vi "Display_ShowGameScreen.vi"(2 "Player":T1) -> ()   [LabVIEW 2018]
uses:
  TypDefs/Player_Enum.ctl
  <vilib>/Platform/TimedLoop/XDataNode/timing_clust.ctl
  <vilib>/Platform/TimedLoop/XDataNode/nitl_modes.ctl
  <vilib>/Platform/TimedLoop/XDataNode/wakeup.ctl
  <vilib>/rvi/Emulation/niFpgaSctlEmulationGetInTimedLoop.vi
  <vilib>/rvi/Emulation/niFpgaEmulationReportErrorSimple.vi
  <vilib>/rvi/Emulation/niFpgaGetClockAttributes.vi
  <vilib>/rvi/Emulation/niFpgaCriticalErrorInLSC.vi
  Control/Global_GameOver.vi
  <vilib>/Platform/TimedLoop/XDataNode/XDataNode.xnode
  <vilib>/Platform/TimedLoop/XDataNode/XDNodeRunTimeDep.lvlib
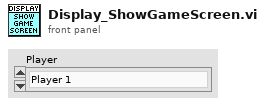
[diagram p1: front panel]
types:
  T1 = typedef "Player_Enum.ctl" = enum16{"Player 1", "Player 2"}
  T2 = typedef "XDNodeRunTimeDep.lvlib/timing_clust.ctl" = cluster{"Expected End [f-1]":u64, "Actual End [f-1]":u64, "Finished Late? [f-1]":bool, "Expected End [i-1]":u64, "Actual End [i-1]":u64, "Finished Late? [i-1]":bool, "Expected Start [i]":u64, "Actual Start [i]":u64, "Expected Start [f]":u64, "Actual Start [f]":u64, "Source Name":string, "Structure Name":string, "Period":i64, "Deadline":i64, "Offset":i64, "Start":i64, "Priority":i32, "Timeout":i32, "Mode":T3, "Wakeup Reason":T4, "Error":errorcluster, "Source Type":string, "Secondary Source Type":string, "Global End Time":u64, "Global Start Time":u64, "Frame Duration":u64, "Iteration Duration":u64, "Assigned CPU":i32, "I/O Scan Engine Mode":u32}
  T3 = typedef "XDNodeRunTimeDep.lvlib/nitl_modes.ctl" = enum32{"No Change", "Process missed periods, maintain original phase", "Discard missed periods, maintain original phase", "Process missed periods, ignore original phase", "Discard missed periods, ignore original phase"}
  T4 = typedef "XDNodeRunTimeDep.lvlib/wakeup.ctl" = enum32{"Normal", "Aborted", "Asynchronous wakeup", "Timing source error", "Timed loop error", "Timeout"}
  T5 = typedef "ActivePixel_Cluster.ctl" = cluster{"h_pixel":i16, "v_pixel":i16}
  T6 = typedef "ActiveTile_Cluster.ctl" = cluster{"h_tile":i16, "v_tile":i16}
  T7 = typedef "Tile_Enum.ctl" = enum8{"Empty", "Snake1_HeadPointingUp", "Snake1_HeadPointingDown", "Snake1_HeadPointingLeft", "Snake1_HeadPointingRight", "Snake1_DeadPointingUp", "Snake1_DeadPointingDown", "Snake1_DeadPointingLeft", "Snake1_DeadPointingRight", "Snake1_TailPointingUp", "Snake1_TailPointingDown", "Snake1_TailPointingLeft", "Snake1_TailPointingRight", "Snake1_Horizontal", "Snake1_Vertical", "Snake1_UpperLeftCorner", "Snake1_UpperRightCorner", "Snake1_LowerLeftCorner", "Snake1_LowerRightCorner", "Snake2_HeadPointingUp", "Snake2_HeadPointingDown", "Snake2_HeadPointingLeft", "Snake2_HeadPointingRight", "Snake2_DeadPointingUp", "Snake2_DeadPointingDown", "Snake2_DeadPointingLeft", "Snake2_DeadPointingRight", "Snake2_TailPointingUp", "Snake2_TailPointingDown", "Snake2_TailPointingLeft", "Snake2_TailPointingRight", "Snake2_Horizontal", "Snake2_Vertical", "Snake2_UpperLeftCorner", "Snake2_UpperRightCorner", "Snake2_LowerLeftCorner", "Snake2_LowerRightCorner", "Wall_Horizontal", "Wall_Vertical", "Wall_UpperLeftCorner", "Wall_UpperRightCorner", "Wall_LowerLeftCorner", "Wall_LowerRightCorner", "Pickup_SpeedUp", "Pickup_Stop", "Pickup_Item1", "Pickup_Item2", "Pickup_Item3", "Pickup_Item4", "Pickup_Item5", "Pickup_Item6"}
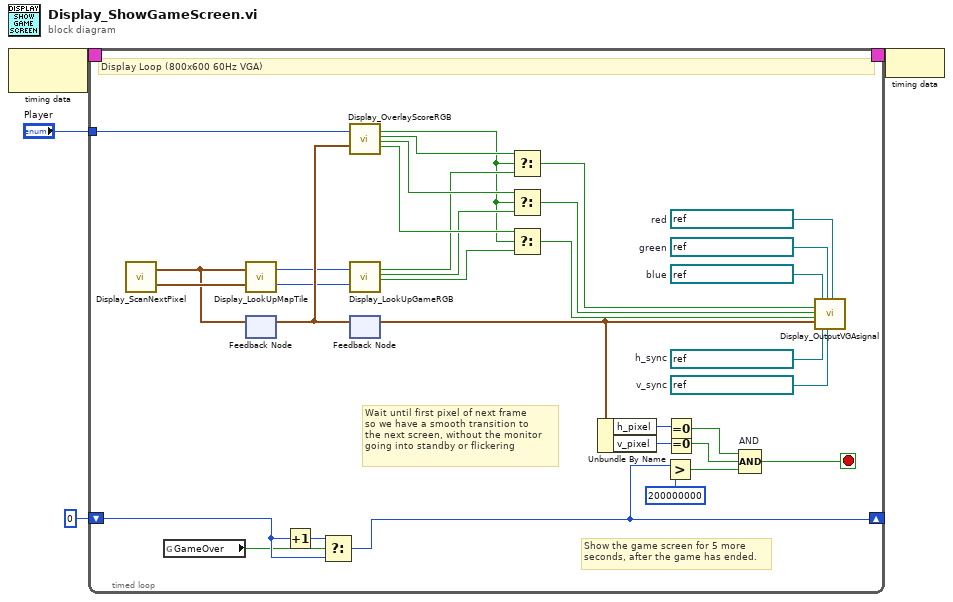
[diagram p0: block diagram]
diagram:
  n1 = node-c288() -> (w4:T2)  [unwired: 1 in]
  n2 = timed-loop {
    timing: w4 -> [_]
    timing-out: [_] -> w3
    shift-right: [w21] -> _
    shift-left: u32 0 -> [w25]
    tunnel: "Player" -> [w17]
    stop <- w26 stop-if-true
    w37 = refnum<k21> "ConnectorC/DIO0"  # red
    w36 = refnum<k21> "ConnectorC/DIO1"  # green
    w35 = refnum<k21> "ConnectorC/DIO2"  # blue
    w33 = refnum<k21> "ConnectorC/DIO4"  # v_sync
    w34 = refnum<k21> "ConnectorC/DIO3"  # h_sync
    # "Show the game screen for 5 more\nseconds, after the game has ended."
    # "Wait until first pixel of next frame\nso we have a smooth transition to\nthe next screen, without the monitor\ngoing into standby or flickering"
    # "Display Loop (800x600 60Hz VGA)"
    n3 = call "Display_ScanNextPixel.vi"() -> ("ActivePixel"=w19:T5, "ActiveTile"=w32:T6)  [unwired: 18 in]
    n4 = global read "Global_GameOver.vi" "GameOver"() -> (w23:bool)
    n5 = call "Display_LookUpMapTile.vi"("ActivePixel"=w19, "ActiveTile"=w32) -> ("ActiveTile"=w6:T7, "TilePixelOffset"=w5:i16)  [unwired: 16 in]
    n6 = feedback #1() -> (w18:T5)  [unwired: 1 in]
    n7 = feedback-in #1(w19) -> ()
    n8 = Increment(x=w25) -> (x+1=w24:u32)
    n9 = Select(t=w24, s=w23, f=w25) -> (s? t:f=w21:u32)
    n10 = call "Display_OverlayScoreRGB.vi"("Player"=w17, "ActivePixel"=w18) -> ("Draw"=w7:bool, "Red"=w16:bool, "Green"=w15:bool, "Blue"=w14:bool)  [unwired: 14 in]
    n11 = call "Display_LookUpGameRGB.vi"("ActiveTile"=w6, "TilePixelOffset"=w5) -> ("Red"=w13:bool, "Green"=w12:bool, "Blue"=w11:bool)  [unwired: 15 in]
    n12 = feedback #2() -> (w31:T5)  [unwired: 1 in]
    n13 = feedback-in #2(w18) -> ()
    n14 = Select(t=w16, s=w7, f=w13) -> (s? t:f=w10:bool)
    n15 = Select(t=w15, s=w7, f=w12) -> (s? t:f=w9:bool)
    n16 = Select(t=w14, s=w7, f=w11) -> (s? t:f=w8:bool)
    n17 = Unbundle By Name(w31) -> ("h_pixel"=w30:i16, "v_pixel"=w29:i16)
    n18 = Greater?(x=w21, y=u32 200000000) -> (0:w22:bool)
    n19 = Equal To 0?(x=w30) -> (x = 0?=w28:bool)
    n20 = Equal To 0?(x=w29) -> (x = 0?=w27:bool)
    n21 = Compound Arithmetic op=AND "AND"(w28, w27, w22) -> (w26:bool)
    n22 = call "Display_OutputVGAsignal.vi"("Red"=w10, "Green"=w9, "Blue"=w8, "ActivePixel"=w31, "Blue [FPGA DO]"=w35, "h_sync [FPGA DO]"=w34, "Green  [FPGA DO]"=w36, "v_sync [FPGA DO]"=w33, "Red  [FPGA DO]"=w37) -> ()  [unwired: 11 in]
  }
  n23 = node-c288(w3) -> ()
